vi "Check if String Valid File Name (SubVI).vi"(0 "String IN":string) -> (4 "String OUT":string)   [LabVIEW 2012]
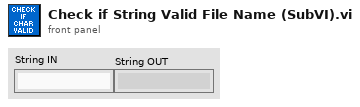
[diagram p1: front panel]
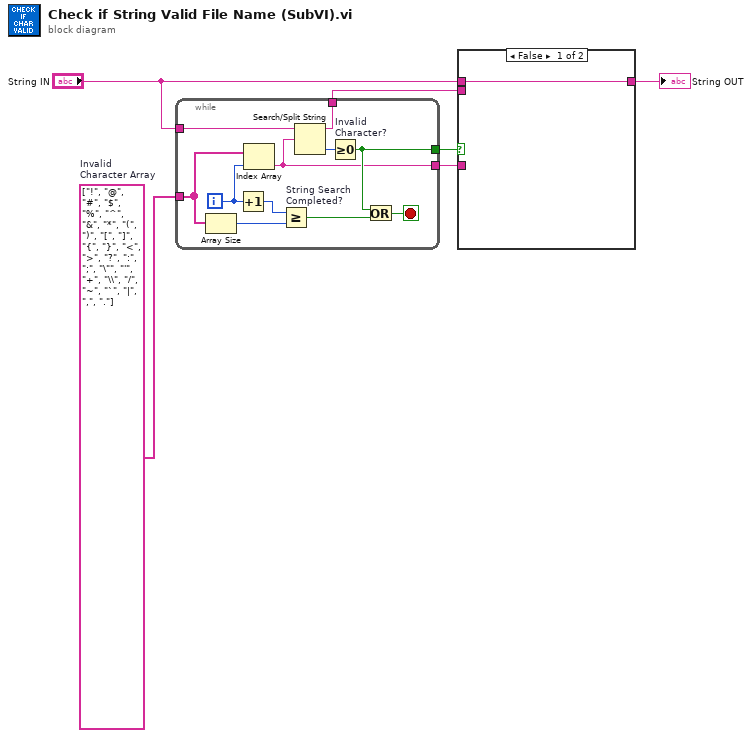
[diagram p0: block diagram]
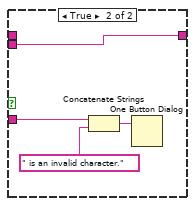
[diagram p2: hidden frame]
diagram:
  w3 = string[] ["!", "@", "#", "$", "%", "^", "&", "*", "(", ")", "[", "]", "{", "}", "<", ">", "?", ":", ";", "\"", "'", "+", "\\", "/", "~", "`", "|", ",", "."]  # Invalid Character Array
  n1 = while {
    tunnel: w3 -> [w16]
    tunnel: [w9] -> w2
    tunnel: "String IN" -> [w13]
    tunnel: [w8] -> w6
    tunnel: [w7] -> w1
    i -> [w12]
    stop <- w15 stop-if-true
    n2 = Array Size(array=w16) -> (size(s)=w17:i32)
    n3 = Increment(x=w12) -> (x+1=w11:i32)
    n4 = Index Array(array=w16, index=w12) -> (element=w8:string)
    n5 = Greater Or Equal? "String Search\nCompleted?"(x=w11, y=w17) -> (x >= y?=w14:bool)
    n6 = Search/Split String(string=w13, search string/char (-)=w8) -> (substring before match=w7:string, offset of match=w10:i32)  [unwired: 1 in, 1 out]
    n7 = Greater Or Equal To 0? "Invalid\nCharacter?"(x=w10) -> (x >= 0?=w9:bool)
    n8 = Or(x=w9, y=w14) -> (x .or. y?=w15:bool)
  }
  n9 = case shown="False" w2 {
    tunnel: "String IN" -> [w18 _]
    tunnel: [w18 w19] -> w5
    tunnel: w6 -> [_ w22]
    tunnel: w1 -> [_ w19]
    frame False {
    }
    frame True {
      n10 = Concatenate Strings(w22, " is an invalid character.") -> (w20:string)
      n11 = One Button Dialog(message=w20) -> ()  [unwired: 1 in, 1 out]
    }
  }
  "String OUT" <- w5
